vi "Write App DAQ Settings File--0.vi"(8 "error in (no error)":errorcluster, 10 "Configuration":T3, 11 "SettingsFolder":path) -> (0 "error out":errorcluster, 3 "SettingsFolder out":path)   [LabVIEW 2017]
doc: "Writes file: \"IOConfig.ini\" at \"ConfigFolder\" folder."
uses:
  <vilib>/Utility/config.llb/NI_LVConfig.lvlib
  DataTypes/TD AI InstSettings--cluster.ctl
  Process/ProcessSupport/TD SimAI Ranges--cluster.ctl
panel:
  # "NOTE: This utility is only used during development\nfor debugging DAQ class."
  # "Writes file: \"Settings.ini\"\nat \"SettingsFolder\" folder."
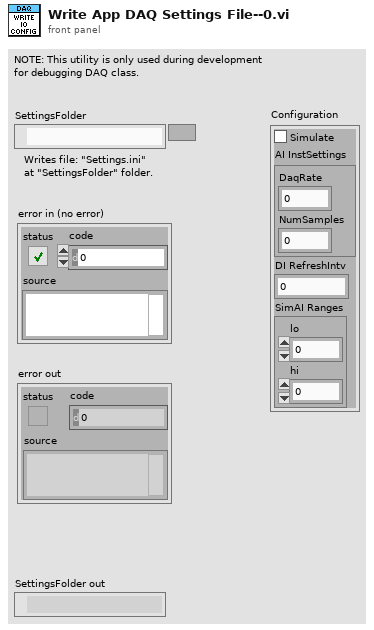
[diagram p1: front panel]
types:
  T1 = typedef "DAQ.lvclass/TD AI InstSettings--cluster.ctl" = cluster{"DaqRate":dbl, "NumSamples":i32}
  T2 = typedef "DAQ.lvclass/TD SimAI Ranges--cluster.ctl" = cluster{"lo":dbl, "hi":dbl}
  T3 = cluster{"Simulate":bool, "AI InstSettings":T1, "DI RefreshIntv":i32, "SimAI Ranges":T2}
  T4 = typedef "NI_LVConfig.lvlib/Config Data RefNum.ctl" = refnum<k1>
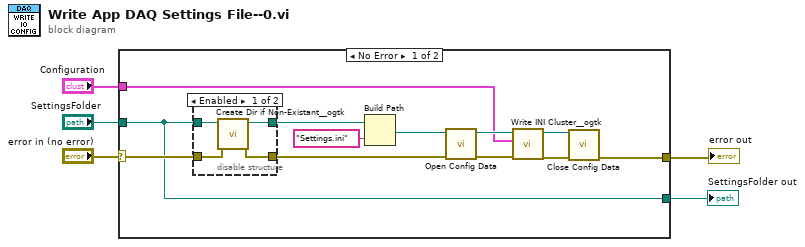
[diagram p0: block diagram]
diagram:
  n1 = case shown="No Error" "error in (no error)" {
    selector: "error in (no error)" -> [w9 w25]
    tunnel: "Configuration" -> [w13 _]
    tunnel: "SettingsFolder" -> [w6 w24]
    tunnel: [w10 w25] -> w3
    tunnel: [w6 w24] -> w1
    frame No Error {
      n2 = disable-structure shown="Enabled" {
        disable-tunnel: w6 -> [w21 w23]
        disable-tunnel: w9 -> [w20 w22]
        disable-tunnel: [w19 w22] -> w8
        disable-tunnel: [w18 w23] -> w7
        frame Enabled {
          n3 = call <userlib>:"Create Dir if Non-Existant__ogtk.vi"("error in (no error)"=w20, "Directory Path"=w21) -> ("error out"=w19:errorcluster, "dup Directory Path"=w18:path)  [unwired: 7 in, 1 out]
        }
        frame Disabled {
        }
      }
      n4 = Build Path(base path=w7, name or relative path="Settings.ini") -> (appended path=w11:path)
      n5 = call <vilib>:"Open Config Data.vi"("error in (no error)"=w8, "configuration file path"=w11) -> ("error out"=w14:errorcluster, "refnum"=w15:T4)  [unwired: 7 in, 1 out]
      n6 = call <userlib>:"Write INI Cluster__ogtk.vi"("error in (no error)"=w14, "INI Fomatted Cluster"=w13, "refnum"=w15) -> ("error out"=w16:errorcluster, "dup refnum"=w17:T4)  [unwired: 7 in]
      n7 = call <vilib>:"Close Config Data.vi"("error in (no error)"=w16, "refnum"=w17) -> ("error out"=w10:errorcluster)  [unwired: 8 in, 1 out]
    }
    frame Error {
    }
  }
  "error out" <- w3
  "SettingsFolder out" <- w1
